vi "Begin.vi"(8 "error in":errorcluster) -> (0 "error out":errorcluster)   [LabVIEW 2016]
doc: "Called before other user functions, this VI can be used to open I/O refnums, load in file data, and do general program initialization. Notice that the <B>error out</B> terminal is simply used for data flow. Wiring it to other structures or subVIs ensures that this VI runs first."
uses:
  <vilib>/Rock Robotics/WPI/DriverStation/WPI_DriverStationRobotMode2.ctl
  <vilib>/Rock Robotics/WPI/Joystick/WPI_JoystickDeviceEnum.ctl
  Robot Global Data.vi
  <vilib>/Rock Robotics/Network Tables/NT Write String Array.vi
  <vilib>/Rock Robotics/WPI/Utilities/WPI_GetSetVariantRefNum.vi
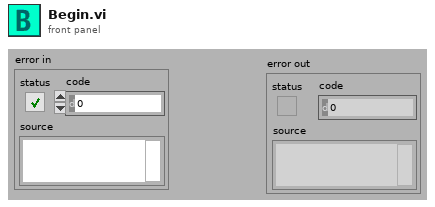
[diagram p1: front panel]
types:
  T1 = typedef "WPI_JoystickDeviceEnum.ctl" = enum16{"USB 0", "USB 1", "USB 2", "USB 3", "USB 4", "USB 5"}
  T2 = typedef "WPI_DriverStationRobotMode2.ctl" = enum16{"Autonomous Disabled", "Autonomous Enabled", "Teleop Disabled", "Teleop Enabled", "Disconnected", "Finish", "Test Disabled", "Test Enabled", "Emergency Stopped"}
  T3 = typedef "WPI_JoystickDevRef.ctl" = cluster{"Device":T1}
  T4 = typedef "WPI_CompressorDevRef.ctl" = cluster{"DevStatus":errorcluster, "Pneumatics Control Module":u8}
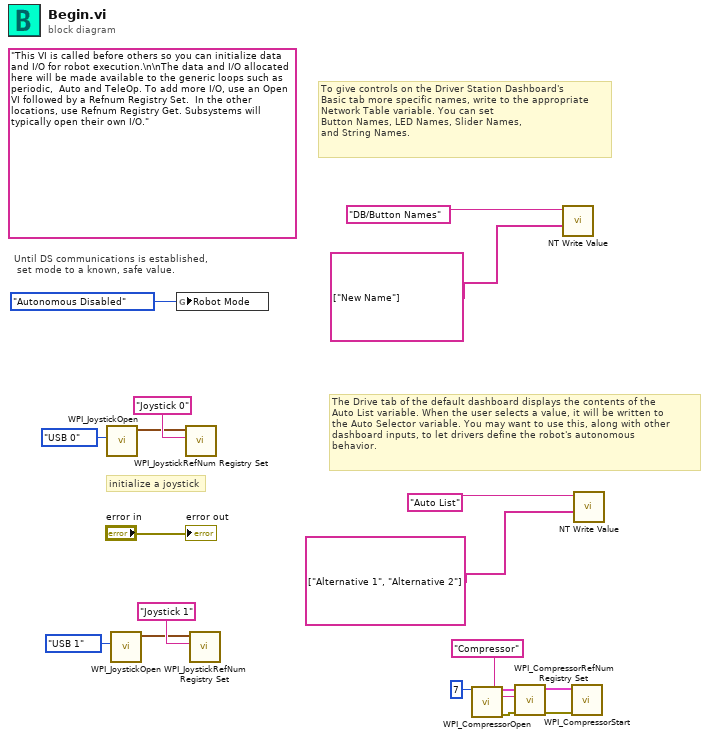
[diagram p0: block diagram]
diagram:
  (unwired) "This VI is called before others so you can initialize data and I/O for robot execution.\n\nThe data and I/O allocated here will be made available to the generic loops such as periodic,  Auto and TeleOp. To add more I/O, use an Open VI followed by a Refnum Registry Set.  In the other locations, use Refnum Registry Get. Subsystems will typically open their own I/O."
  # "The Drive tab of the default dashboard displays the contents of the\nAuto List variable. When the user selects a value, it will be written to\nthe Auto Selector variable. You may want to use this, along with other\ndashboard inputs, to let drivers define the robot's autonomous\nbehavior."
  # "To give controls on the Driver Station Dashboard's\nBasic tab more specific names, write to the appropriate\nNetwork Table variable. You can set\nButton Names, LED Names, Slider Names,\nand String Names."
  # "initialize a joystick"
  # "Until DS communications is established,\n set mode to a known, safe value."
  n1 = call <vilib>:"WPI_JoystickOpen.vi"("JoystickDevice"=WPI_JoystickDeviceEnum."USB 0") -> ("JoystickDevRef"=w16:T3)  [unwired: 10 in]
  n2 = call <vilib>:"WPI_JoystickOpen.vi"("JoystickDevice"=WPI_JoystickDeviceEnum."USB 1") -> ("JoystickDevRef"=w8:T3)  [unwired: 10 in]
  n3 = global write "Robot Global Data.vi" "Robot Mode"(WPI_DriverStationRobotMode2."Autonomous Disabled" ("Robot Mode")) -> ()
  n4 = call <vilib>:"WPI_JoystickRefNum Registry Set.vi"("refnum name"="Joystick 0", "JoystickDevRef"=w16) -> ()  [unwired: 8 in, 2 out]
  n5 = call <vilib>:"WPI_JoystickRefNum Registry Set.vi"("refnum name"="Joystick 1", "JoystickDevRef"=w8) -> ()  [unwired: 8 in, 2 out]
  n6 = call <vilib>:"WPI_CompressorOpen.vi"("Pneumatics Control Module (0)"=u8 7) -> ("CompressorDevRef"=w5:T4, "error out"=w6:errorcluster)  [unwired: 13 in]
  n7 = call <vilib>:"WPI_CompressorRefNum Registry Set.vi"("error in (no error)"=w6, "refnum name"="Compressor", "CompressorDevRef"=w5) -> ("error out"=w3:errorcluster, "CompressorDevRef"=w2:T4)  [unwired: 7 in]
  n8 = call-poly <vilib>:"NT Write Value.vi"("String Array"=string[] ["New Name"], "Name"="DB/Button Names") -> ()  [unwired: 9 in, 1 out]
  n9 = call <vilib>:"WPI_CompressorStart.vi"("error in (no error)"=w3, "CompressorDevRef"=w2) -> ()  [unwired: 8 in, 2 out]
  n10 = call-poly <vilib>:"NT Write Value.vi"("String Array"=string[] ["Alternative 1", "Alternative 2"], "Name"="Auto List") -> ()  [unwired: 9 in, 1 out]
  "error out" <- "error in"
